vi "Set Motor Speed.vi"(8 "error in (no error)":errorcluster, 9 "Speed":u8, 10 "Motor":u16, 11 "Grove I2C L298P Motor Drive in":refnum<class "Grove I2C L298P Motor Drive.lvclass">) -> (0 "error out":errorcluster, 3 "Grove I2C L298P Motor Drive out":refnum<class "Grove I2C L298P Motor Drive.lvclass">)   [LabVIEW 2020, in "CTI-Peripheral.lvlib" / "Grove I2C L298P Motor Drive.lvclass"]
uses:
  Grove I2C L298P Motor Drive.lvclass
  Grove I2C L298P Motor Drive.lvclass/Grove I2C L298P Motor Drive.ctl
  CTI/I2C Connection/I2C Connection.lvclass/I2C Connection.ctl
  CTI/Session/I2C Write Data.vi
  CTI/I2C Connection/I2C Connection.lvclass
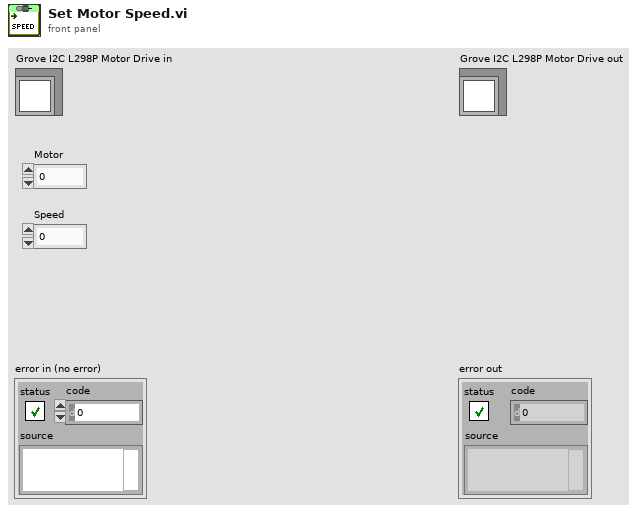
[diagram p1: front panel]
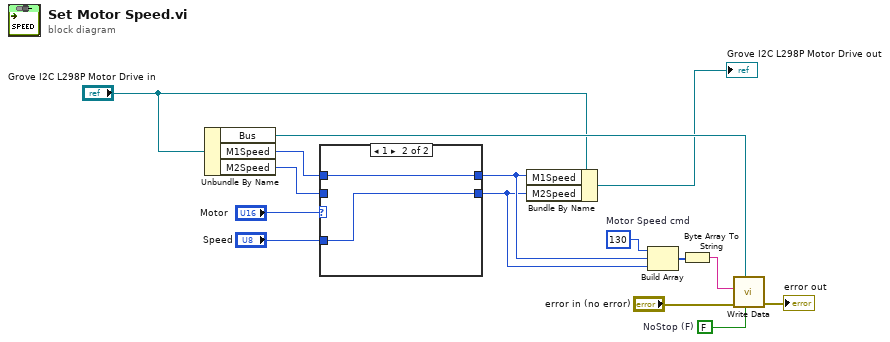
[diagram p0: block diagram]
diagram:
  w12 = u8 130  # Motor Speed cmd
  w13 = FALSE  # NoStop (F)
  n1 = Unbundle By Name("Grove I2C L298P Motor Drive in") -> ("Bus"=w14:refnum<class "I2C Connection.lvclass">, "M1Speed"=w4:u8, "M2Speed"=w3:u8)
  n2 = case shown="1" "Motor" {
    tunnel: "Speed" -> [w17 w18]
    tunnel: w4 -> [_ w19]
    tunnel: w3 -> [w16 _]
    tunnel: [w17 w19] -> w2
    tunnel: [w16 w18] -> w1
    frame 0, Default {
    }
    frame 1 {
    }
  }
  n3 = Bundle By Name(cluster="Grove I2C L298P Motor Drive in", "M1Speed"=w2, "M2Speed"=w1) -> (→"Grove I2C L298P Motor Drive out":refnum<class "Grove I2C L298P Motor Drive.lvclass">)
  n4 = Build Array(w12, w2, w1) -> (w11:u8[])
  n5 = Byte Array To String(unsigned byte array=w11) -> (string=w9:string)
  n6 = call "Write Data.vi"("NoStop (F)"=w13, "I2C Connection"=w14, "error in (no error)"="error in (no error)", "Data"=w9) -> ("error out"=→"error out":errorcluster)  [unwired: 7 in]
